vi "image combine (SubVI).vi"(8 "spacing":i32, 9 "zx":u16[][](array[numeric])=[[5, 5, 5]], 10 "yz":u16[][](array[numeric])=[[3, 3, 3], [3, 3, 3]], 11 "yx":u16[][](array[numeric])=[[1, 1, 2], [1, 1, 2]]) -> (3 "combined":u16[][](array[numeric])=[[1, 1, 2, 3, 3, 3], [1, 1, 2, 3, 3, 3], [5, 5, 5, 0, 0, 0]])   [LabVIEW 2024]
panel:
  out "Intensity Graph":u16[][](graph)
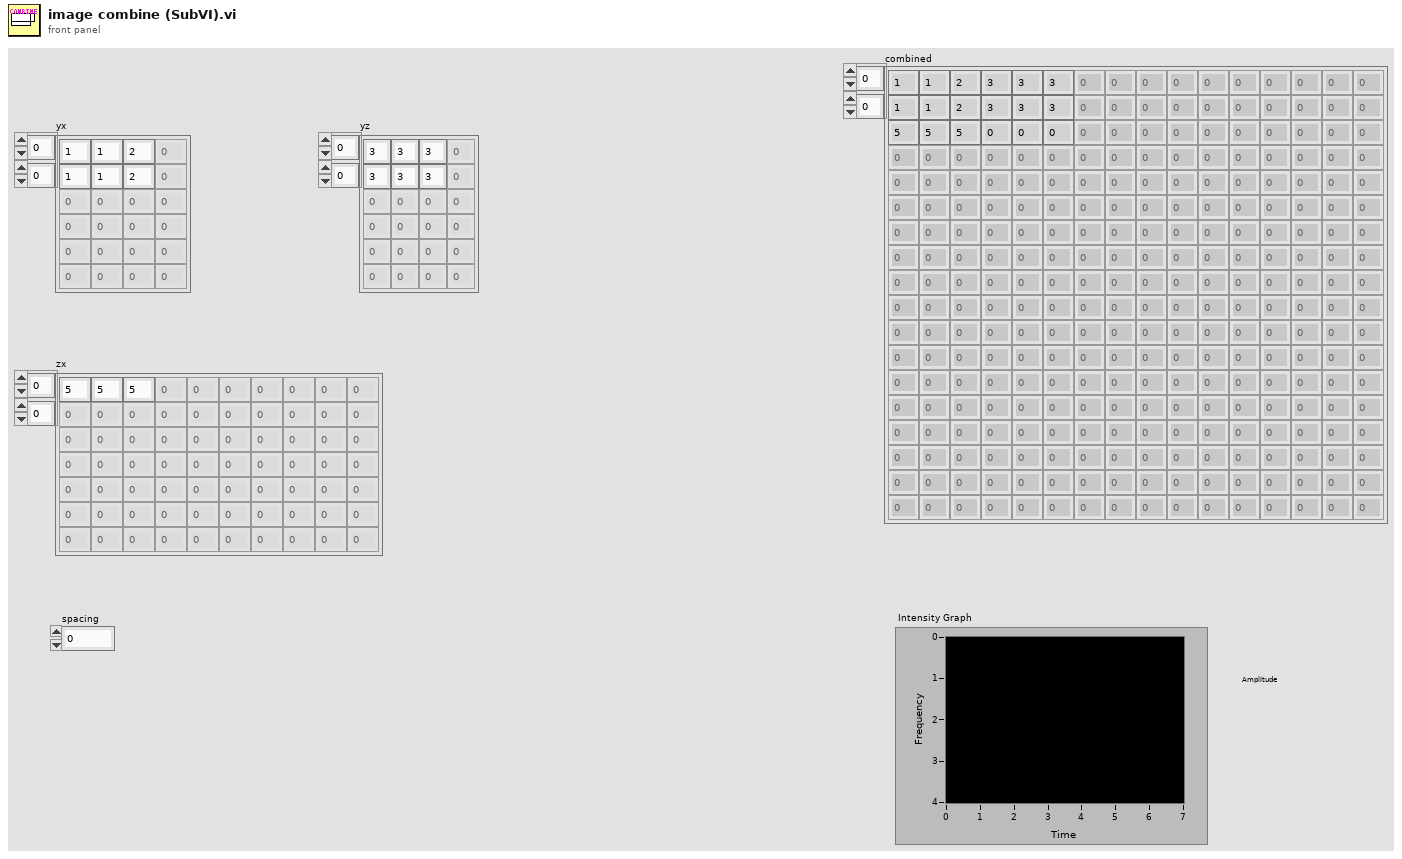
[diagram p1: front panel]
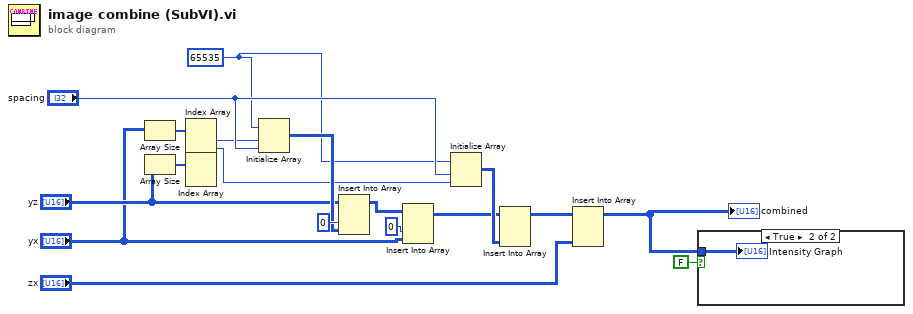
[diagram p0: block diagram]
diagram:
  w4 = u16 65535
  n1 = Array Size(array="yx") -> (size(s)=w15:i32[])
  n2 = Array Size(array="yz") -> (size(s)=w14:i32[])
  n3 = Index Array(array=w15) -> (element #1=w2:i32, element #2=w1:i32)  [unwired: 2 in]
  n4 = Index Array(array=w14) -> ()  [unwired: 2 in, 2 out]
  n5 = Initialize Array(w4, w2, "spacing") -> (w11:u16[][])
  n6 = Insert Into Array(array="yz", index (col)=0 ("disabled index (col)"), new element=w11) -> (w12:u16[][])  [unwired: 1 in]
  n7 = Insert Into Array(array=w12, index (col)=0 ("disabled index (col)"), new element="yx") -> (w7:u16[][])  [unwired: 1 in]
  n8 = Initialize Array(w4, "spacing", w1) -> (w8:u16[][])
  n9 = Insert Into Array(array=w7, new element=w8) -> (w6:u16[][])  [unwired: 2 in]
  n10 = Insert Into Array(array=w6, new element="zx") -> (w17:u16[][])  [unwired: 2 in]
  "combined" <- w17
  n11 = case shown="True" FALSE {
    tunnel: w17 -> [_ w19]
    frame False {
    }
    frame True {
      "Intensity Graph" <- w19
    }
  }
